vi "FG Dispatcher Status.vi"(0 "action (Get)":T1, 5 "UDP port in (0)":u16, 11 "error in":errorcluster) -> (4 "UDP connection ID":refnum<k16>, 6 "UDP port out":u16, 15 "error out":errorcluster)   [LabVIEW 2009, in "AMC.lvlib"]
uses:
  AMC.lvlib
  FG Dispatcher Status Action.ctl
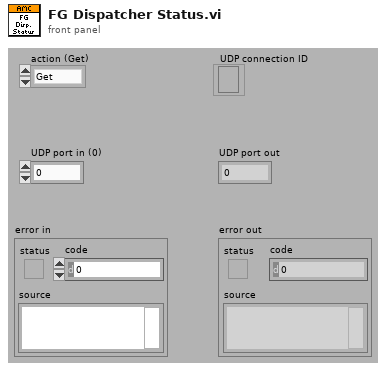
[diagram p1: front panel]
types:
  T1 = typedef "AMC.lvlib/FG Dispatcher Status Action.ctl" = enum16{"Get", "Force Init", "Close"}
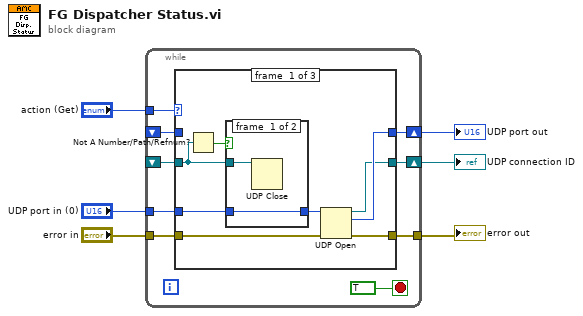
[diagram p0: block diagram]
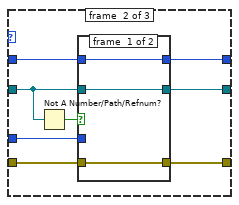
[diagram p3: hidden frame]
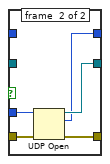
[diagram p4: hidden frame]
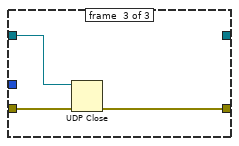
[diagram p5: hidden frame]
diagram:
  n1 = while {
    shift-right: [w14] -> w5
    shift-left: _ -> [w13]
    tunnel: [w12] -> w6
    tunnel: "error in" -> [w11]
    tunnel: "UDP port in (0)" -> [w9]
    tunnel: "action (Get)" -> [w10]
    shift-right: [w8] -> w2
    shift-left: _ -> [w7]
    stop <- TRUE stop-if-true
    n2 = case shown="\"Get\"" w10 {
      tunnel: w9 -> [w17 w34 _]
      tunnel: [w18 w33 _] -> w14
      tunnel: w13 -> [w22 w30 w45]
      tunnel: [w20 w31 w44] -> w12
      tunnel: w11 -> [w21 w32 w43]
      tunnel: [w19 w28 _] -> w8
      tunnel: w7 -> [_ w29 _]
      frame #0 {
        n3 = Not A Number/Path/Refnum?(number/path/refnum=w22) -> (NaN/Path/Refnum?=w23:bool)
        n4 = case shown="False" w23 {
          tunnel: w22 -> [w25 _]
          tunnel: w17 -> [w24 w26]
          tunnel: [w24 w26] -> w16
          frame #0 {
            n5 = UDP Close(connection ID=w25) -> ()  [unwired: 1 in, 2 out]
          }
          frame #1 {
          }
        }
        n6 = UDP Open(8:w21, 11:w16) -> (port=w18:refnum<k16>, 0:w20:errorcluster, 2:w19:u16)  [unwired: 3 out]
      }
      frame #1 {
        n7 = Not A Number/Path/Refnum?(number/path/refnum=w30) -> (NaN/Path/Refnum?=w27:bool)
        n8 = case shown="True" w27 {
          tunnel: w34 -> [_ w39]
          tunnel: [w37 w42] -> w33
          tunnel: w30 -> [w37 _]
          tunnel: w32 -> [w36 w41]
          tunnel: [w36 w40] -> w31
          tunnel: w29 -> [w35 _]
          tunnel: [w35 w38] -> w28
          frame #0 {
          }
          frame #1 {
            n9 = UDP Open(8:w41, 11:w39) -> (port=w42:refnum<k16>, 0:w40:errorcluster, 2:w38:u16)  [unwired: 3 out]
          }
        }
      }
      frame #2 {
        n10 = UDP Close(connection ID=w45, 8:w43) -> (error out=w44:errorcluster)  [unwired: 1 out]
      }
    }
  }
  "UDP connection ID" <- w5
  "error out" <- w6
  "UDP port out" <- w2
